vi "_Global LC Driver.vi"() -> ()   [LabVIEW 2015]
uses:
  Type/_LC Type.ctl
  Type/_LC Command.ctl
  Type/_LcRackType.ctl
panel:
  out "IsSimplcityServer":bool
  in  "ActiveStream#":u8
  out "IsDual":bool
  in  "MethodStream#":u8
  out "RunOrder":i16=1
  in  "SparkParameters":T1={"PlatePosition"=1, "SampleColumn"=97, "TrayType"=3}
  out "Reply":string
  out "LC Error":errorcluster
  in  "RackType":T2 items=["RackSVial"=0, "RackLVial"=1, "RackSPeltier"=2, "RackLPeltier"=3, "RackSingleMTP"=4, "RackDualMTP"=5, "RackLL"=6, "Rack2"=17, "Rack1"=18, "Rack3"=19, "Rack4"=20, "Rack5"=21, "Rack6"=22, "Rack7"=23, "Rack12"=33, "Rack11"=34, "Rack13"=35, "Rack14"=36, "Rack15"=37, "Rack16"=38, "Rack17"=39, "Rack_2010A_15Standard"=49, "Rack_2010A_1Standard"=50, "Rack_2010A_4Standard"=51, "Rack_2010A_MTP96Standard"=52, "Rack_2010A_MTP384Standard"=53, "Rack_2010A_DW96Standard"=54, "Rack_2010A_DW384Standard"=55, "Rack_2010A_15Cooled"=65, "Rack_2010A_1Cooled"=66, "Rack_2010A_4Cooled"=67, "Rack_2010A_MTP96Cooled"=68, "Rack_2010A_MTP384Cooled"=69, "Rack_2010A_DW96Cooled"=70, "Rack_2010A_DW384Cooled"=71, "Rack_20A_RACKCHANGER"=72, "Rack12A"=80, "Rack14A"=81, "Rack8"=82, "Rack9"=83, "Rack10"=84, "Rack14DDW"=85, "Rack5U"=86, "Rack4U"=87, "ControlRack"=119, "RackNone"=136, "RackUnknown"=153]
  in  "InjectionVolume":dbl
  in  "VialNumber":i16
  out "LC Driver Running":bool
  out "Execute LC Command":bool
  out "Parameter":string
  in  "Stream#":u8
  in  "LC Command":T3=enum."Initialize"
  in  "LC Type":T4
  # "(use in send LC Command)"
  # "(use in run engine)"
  # "(used in manual LC control)"
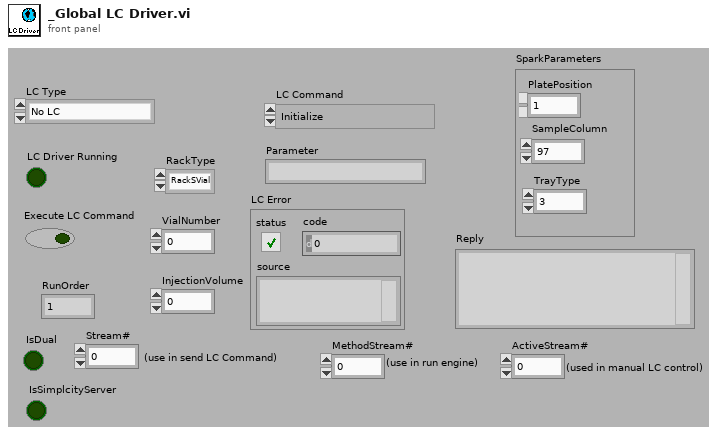
[diagram p1: front panel]
types:
  T1 = cluster{"PlatePosition":u8, "SampleColumn":u8, "TrayType":u8}
  T2 = typedef "_LcRackType.ctl" = i32
  T3 = typedef "_LC Command.ctl" = enum16{"No Command", "Initialize", "Get Configuration", "Get Status", "Get LC Method Contents", "Oven OnOff", "Pump OnOFF", "Rinse Autosampler", "Run Sample", "Set EnvParameters", "Set Method", "Start Equilibration", "Stop Run", "Get LastError", "Clear Error", "Close"}
  T4 = typedef "_LC Type.ctl" = enum16{"No LC", "Spark"}
diagram:
